vi "Format Bool Array Cmd.vi"(4 "Command":T1[](array[typedef])) -> (7 "String":string)   [LabVIEW 2020, in "Volatus.lvlib" / "Module.lvclass"]
uses:
  Module.lvclass
  messages/CmdDigital/Data.ctl
  Module.lvclass/Module.ctl
  lv-vecto/Vecto/Vecto.lvlib
  messages/CmdDigital/CmdDigital.lvlib
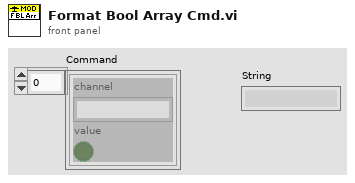
[diagram p1: front panel]
types:
  T1 = typedef "CmdDigital.lvlib/Data.ctl" = cluster{"channel":string, "value":bool}
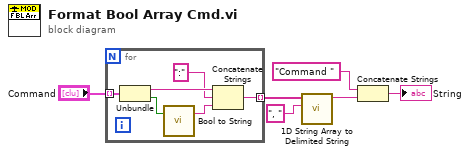
[diagram p0: block diagram]
diagram:
  n1 = for {
    tunnel: "Command" -> [w12] mode=indexing
    tunnel: [w7] -> w5 mode=indexing
    n2 = Unbundle(w12) -> ("channel"=w10:string, "value"=w11:bool)
    n3 = call "Bool to String.vi"("Bool"=w11) -> ("String"=w8:string)  [unwired: 2 in]
    n4 = Concatenate Strings(w10, ":" ("string"), w8) -> (w7:string)
  }
  n5 = call <vilib>:"1D String Array to Delimited String.vi"("delimiter"=", ", "string array"=w5) -> ("delimited string"=w3:string)  [unwired: 9 in]
  n6 = Concatenate Strings("Command " ("string"), w3) -> (→"String":string)
